vi "Arm.vi"(8 "error in (no error)":errorcluster, 11 "GaGe Digitizer in":refnum<class "GaGe Digitizer.lvclass">) -> (0 "error out":errorcluster, 3 "GaGe Digitizer out":refnum<class "GaGe Digitizer.lvclass">)   [LabVIEW 2015, in "GaGe Digitizer.lvclass"]
uses:
  GaGe Digitizer.lvclass
  GaGe Digitizer.lvclass/GaGe Digitizer.ctl
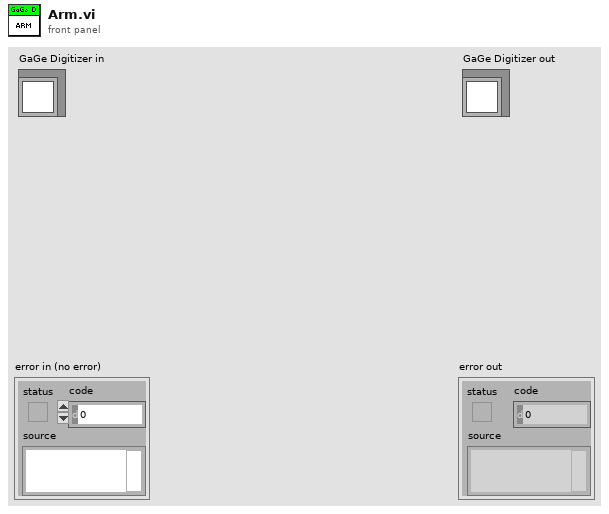
[diagram p1: front panel]
types:
  T1 = cluster{"Handle":u32, "Sample size":u32, "Resolution":i32, "Offset":i32, "Channels":u32, "Boards":u32}
  T2 = typedef "Timing Element.ctl" = cluster{"Data rate":dbl, "Record length":dbl, "Pre-trigger length":dbl, "Ext. clock":bool}
  T3 = cluster{"Range":dbl, "Coupling":enum16{"Single", "Differen"}, "Impedance":dbl}[]
  T4 = cluster{"Device Name":string, "Number of channels":i32, "Device Index":i32, "Device type":enum16{"GaGe", "NI-DAQ", "NI-Scope", "CAMAC", "VXI-1433", "VXI-1437"}, "Total points":i64, "Current position":i64, "Chunk size":i64, "Active":bool, "Oversample by":i32, "Pre-trigger points":i64, "Fast mode":bool}
  T5 = cluster{"Trig. edge":enum16{"Rising", "Falling"}, "Trig. type":enum16{"Reference", "Immediate", "Start"}, "Trig. level":sgl, "Average samples":bool, "Oversample\nto match rates":bool}
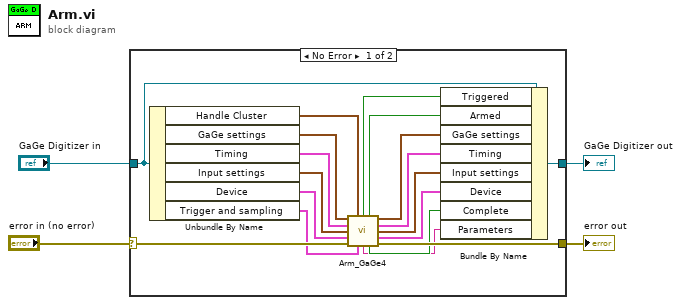
[diagram p0: block diagram]
diagram:
  n1 = case shown="No Error" "error in (no error)" {
    selector: "error in (no error)" -> [w16 w24]
    tunnel: [w15 w24] -> w3
    tunnel: [w13 w23] -> w1
    tunnel: "GaGe Digitizer in" -> [w22 w23]
    frame No Error {
      n2 = Unbundle By Name(w22) -> ("Handle Cluster"=w21:T1, "GaGe settings"=w20:cluster{"Mode":u16}, "Timing"=w19:T2, "Input settings"=w18:T3, "Device"=w17:T4, "Trigger and sampling"=w14:T5)
      n3 = call "Arm_GaGe4.vi"("GaGe settings"=w20, "Handle Cluster"=w21, "Timing"=w19, "Input settings"=w18, "Device"=w17, "error in (no error)"=w16, "Trigger and sampling"=w14) -> ("Triggered"=w8:bool, "Armed"=w9:bool, "GaGe settings out"=w12:cluster{"Mode":u16}, "Timing"=w11:T2, "Input settings out"=w10:T3, "Device out"=w7:T4, "Parameters"=w5:string, "Complete"=w6:bool, "error out"=w15:errorcluster)
      n4 = Bundle By Name(cluster=w22, "Triggered"=w8, "Armed"=w9, "GaGe settings"=w12, "Timing"=w11, "Input settings"=w10, "Device"=w7, "Complete"=w6, "Parameters"=w5) -> (w13:refnum<class "GaGe Digitizer.lvclass">)
    }
    frame Error {
    }
  }
  "error out" <- w3
  "GaGe Digitizer out" <- w1
